vi "CRYGet Spectrum Curve.vi"(9 "Unit Info In":T5={"Y unit In"="dB", "dB ref In"=1.0, "Y unit Out"="dB", "dB ref Out"=1.0, "Y unit Curve"="dB", "dB ref Curve"=1.0, "Y data  Curve"=0, "Y data Time"=0}, 10 "Additive Info":T3) -> (1 "Display Array":T4(array[cluster]), 2 "Unit Info Out":T2[](array[typedef]), 3 "Curve Info Array Out":T1)   [LabVIEW 2013]
uses:
  Typedef Control/CRYUnit Info Cluster.ctl
  Typedef Control/CRYUnit Info Out Cluster.ctl
  Typedef Control/CRYAnalysis CurveName Cluster.ctl
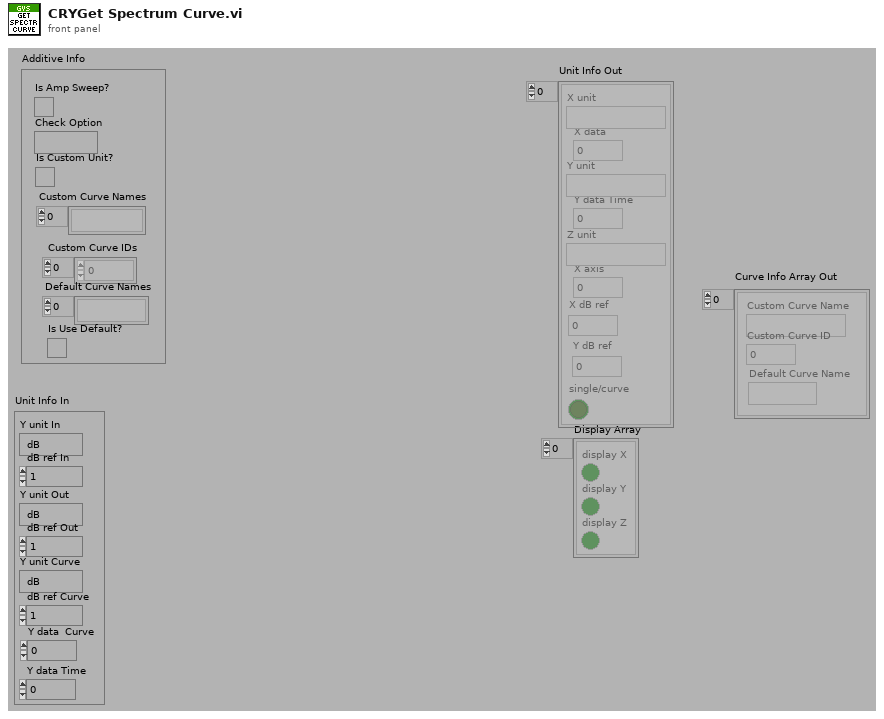
[diagram p1: front panel]
types:
  T1 = typedef "CRYAnalysis CurveName Cluster.ctl" = cluster{"Custom Curve Name":string, "Custom Curve ID":i32, "Default Curve Name":string}[]
  T2 = typedef "CRYUnit Info Out Cluster.ctl" = cluster{"X unit":string, "X data":u16, "Y unit":string, "Y data Time":u16, "Z unit":string, "X axis":u16, "X dB ref":dbl, "Y dB ref":dbl, "single/curve":bool}
  T3 = cluster{"Is Amp Sweep?":bool, "Check Option":string, "Is Custom Unit?":bool, "Custom Curve Names":string[], "Custom Curve IDs":i32[], "Default Curve Names":string[], "Is Use Default?":bool}
  T4 = cluster{"display X":bool, "display Y":bool, "display Z":bool}[]
  T5 = typedef "CRYUnit Info Cluster.ctl" = cluster{"Y unit In":string, "dB ref In":dbl, "Y unit Out":string, "dB ref Out":dbl, "Y unit Curve":string, "dB ref Curve":dbl, "Y data  Curve":u16, "Y data Time":u16}
  T6 = cluster{"display X":bool, "display Y":bool, "display Z":bool}
  T7 = enum32{"English", "Chinese", "Korean", "Japanese", "Russian", "Chinese traditional"}
  T8 = cluster{"Y unit Out":string, "dB":u16, "Y unit Curve":string, "Y data  Curve":u16, "Y unit Curve":string, "Lin":u16, "dB ref Out":dbl, "dB ref Curve":dbl, "display X":bool}
  T9 = cluster{"Y unit Out":string, "dB":u16, "Y unit Curve":string, "Y data  Curve":u16, "Y unit Curve":string, "Lin":u16, "dB ref Out":dbl, "dB ref Curve":dbl, "display X":bool}[]
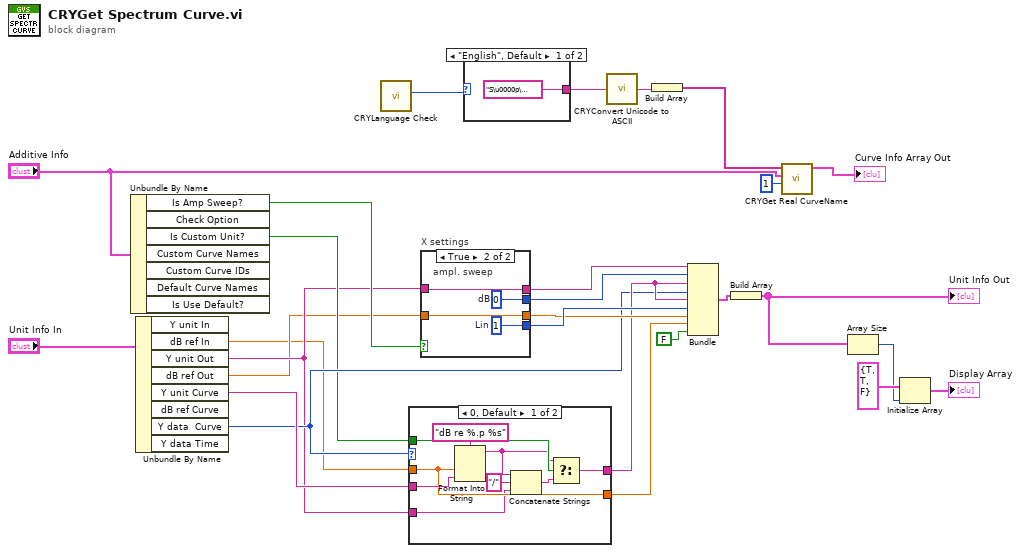
[diagram p0: block diagram]
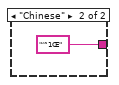
[diagram p2: hidden frame]
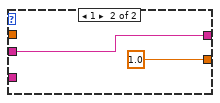
[diagram p3: hidden frame]
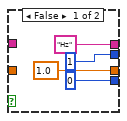
[diagram p4: hidden frame]
diagram:
  n1 = Unbundle By Name("Additive Info") -> ("Is Amp Sweep?"=w24:bool, "Is Custom Unit?"=w12:bool)  [unwired: 5 out]
  n2 = Unbundle By Name("Unit Info In") -> ("dB ref In"=w6:dbl, "Y unit Out"=w11:string, "dB ref Out"=w7:dbl, "Y unit Curve"=w16:string, "Y data  Curve"=w13:u16)  [unwired: 3 out]
  n3 = call "CRYLanguage Check.vi"() -> ("Language"=w2:T7)  [unwired: 10 in, 1 out]
  n4 = case shown="0, Default" w13 {
    tunnel: [w28 w37] -> w14
    tunnel: w6 -> [w34 _]
    tunnel: w16 -> [w35 w37]
    tunnel: [w34 1.0 ("dB ref Curve")] -> w15
    tunnel: w12 -> [w33 _]
    tunnel: w11 -> [w30 _]
    frame 0, Default {
      n5 = Format Into String(format string="dB re %.p %s", w34, w35) -> (resulting string=w32:string)  [unwired: 2 in, 1 out]
      n6 = Concatenate Strings(w32, "/" ("string"), w30) -> (w29:string)
      n7 = Select(t=w32, s=w33, f=w29) -> (s? t:f=w28:string)
    }
    frame 1 {
    }
  }
  n8 = case "X settings" shown="True" w24 {
    tunnel: ["Hz" ("X unit") w44] -> w23
    tunnel: [u16 1 ("Y data") w45] -> w22
    tunnel: [1.0 ("X dB ref") w43] -> w20
    tunnel: [u16 0 ("X axis") w46] -> w21
    tunnel: w11 -> [_ w44]
    tunnel: w7 -> [_ w43]
    frame False {
    }
    frame True {
      w45 = u16 0  # dB
      w46 = u16 1  # Lin
      # "ampl. sweep"
    }
  }
  n9 = case shown="\"English\", Default" w2 {
    tunnel: ["S\u0000p\u0000e\u0000c\u0000t\u0000r\u0000u\u0000m\u0000" ("Unicode") "‘˜1Œ" ("Unicode")] -> w4
    frame "English", Default {
    }
    frame "Chinese" {
    }
  }
  n10 = call "CRYConvert Unicode to ASCII.vi"("Unicode"=w4) -> ("ASCII"=w3:string)  [unwired: 4 in]
  n11 = Build Array(w3) -> (w5:string[])
  n12 = Bundle("Y unit Out"=w23, "dB"=w22, "Y unit Curve"=w14, "Y data  Curve"=w13, "Y unit Curve"=w14, "Lin"=w21, "dB ref Out"=w20, "dB ref Curve"=w15, "display X"=FALSE) -> (w18:T8)  [unwired: 1 in]
  n13 = Build Array(w18) -> (w17:T9)
  "Unit Info Out" <- w17
  n14 = call "CRYGet Real CurveName.vi"("Key No"=1, "Additive Info"="Additive Info", "CurveArrayByType"=w5) -> ("Curve Info Array Out"=→"Curve Info Array Out":T1)  [unwired: 8 in]
  n15 = Array Size(array=w17) -> (size(s)=w26:i32)
  n16 = Initialize Array(T6 {"display X"=TRUE, "display Y"=TRUE, "display Z"=FALSE}, w26) -> (→"Display Array":T4)
